vi "EminemGetCommandReady.vi"() -> (0 "BoxCommandReady":bool)   [LabVIEW 2023]
uses:
  EminemGlobals.vi
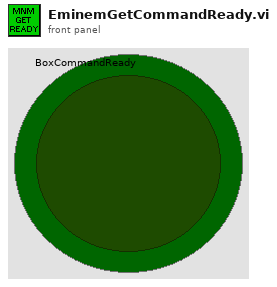
[diagram p1: front panel]
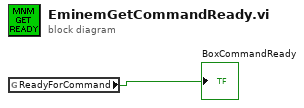
[diagram p0: block diagram]
diagram:
  n1 = global read "EminemGlobals.vi" "ReadyForCommand"() -> (→"BoxCommandReady":bool)
